vi "Channel Basics Lesson 8.vi"() -> ()   [LabVIEW 2019]
doc: "This VI demonstrates that channels can create cycles among nodes, unlike regular dataflow wires."
uses:
  <extravilib>/ChannelInstances/One Element Stream-i32/Read With Abort.vi
  <extravilib>/ChannelInstances/One Element Stream-i32/Write With Abort.vi
  <extravilib>/ChannelInstances/One Element Stream-i32/Instantiate.vi
  <extravilib>/ChannelInstances/One Element Stream-i32/EndpointRead.vi
  <extravilib>/ChannelInstances/One Element Stream-i32/Endpoint.vi
  <extravilib>/ChannelInstances/One Element Stream-i32.lvlib
panel:
  out "gamma":i32
  out "beta":i32
  out "alpha":i32
  # "Overview: This VI demonstrates that channels can create cycles among nodes, unlike regular dataflow wires.\n\nInstructions:\n1. Open the block diagram. Review the lessons presented there.\n2. Run the VI and observe the values of alpha, beta, and gamma show the results of the integer being passed from loop to loop."
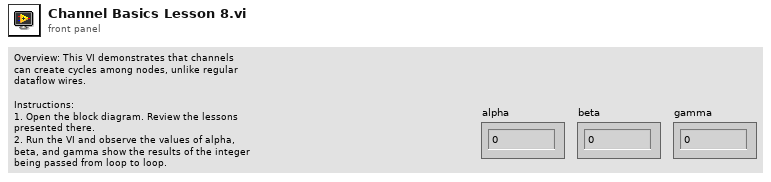
[diagram p1: front panel]
types:
  T1 = typedef "One Element Stream-i32.lvlib/)Channel.ctl" = refnum<queue>
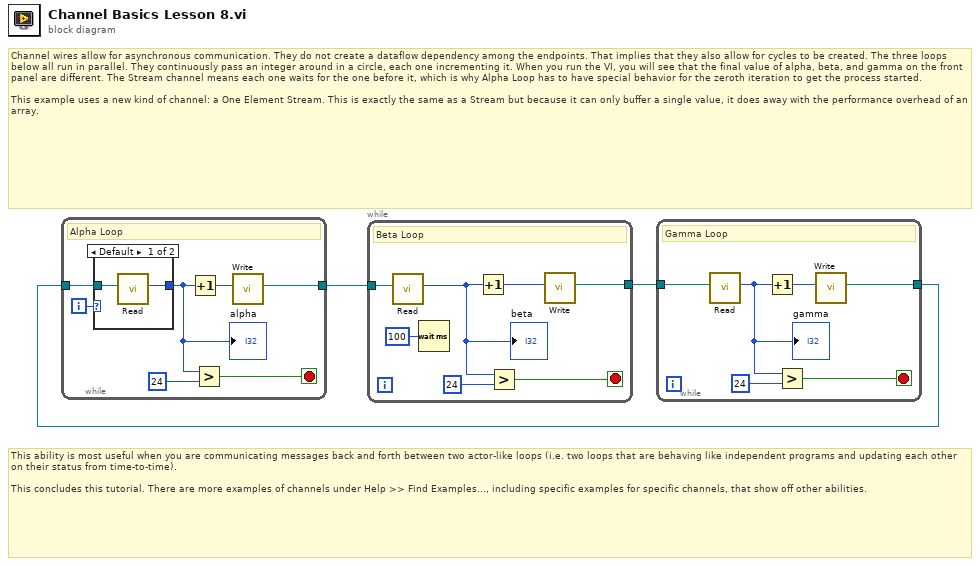
[diagram p0: block diagram]
diagram:
  # "This ability is most useful when you are communicating messages back and forth between two actor-like loops (i.e. two loops that are behaving like independent programs and updating each other on their status from time-to-time).\n\nThis concludes this tutorial. There are more examples of channels under Help >> Find Examples..., including specific examples for specific channels, that show off other abilities."
  # "Channel wires allow for asynchronous communication. They do not create a dataflow dependency among the endpoints. That implies that they also allow for cycles to be created. The three loops below all run in parallel. They continuously pass an integer around in a circle, each one incrementing it. When you run the VI, you will see that the final value of alpha, beta, and gamma on the front panel are different. The Stream channel means each one waits for the one before it, which is why Alpha Loop has to have special behavior for the zeroth iteration to get the process started.\n\nThis example uses a new kind of channel: a One Element Stream. This is exactly the same as a Stream but because it can only buffer a single value, it does away with the performance overhead of an array."
  n1 = while {
    tunnel: [w4] -> w1
    tunnel: w2 -> [w10]
    i -> [w6]
    stop <- w7 stop-if-true
    # "Alpha Loop"
    n2 = case shown="Default" w6 {
      tunnel: w10 -> [w12 _]
      tunnel: [w11 _] -> w9
      frame Default {
        n3 = call <extravilib>:"Read.vi"("channel"=w12) -> ("element"=w11:i32)  [unwired: 7 in, 3 out]
      }
      frame 0 {
      }
    }
    "alpha" <- w9
    n4 = Increment(x=w9) -> (x+1=w5:i32)
    n5 = Greater?(x=w9, y=24) -> (0:w7:bool)
    n6 = call <extravilib>:"Write.vi"("element"=w5) -> ("channel"=w4:T1)  [unwired: 9 in, 1 out]
  }
  n7 = while {
    tunnel: w1 -> [w14]
    tunnel: [w15] -> w3
    stop <- w18 stop-if-true
    # "Beta Loop"
    n8 = call <extravilib>:"Read.vi"("channel"=w14) -> ("element"=w13:i32)  [unwired: 7 in, 3 out]
    "beta" <- w13
    n9 = Wait (ms)(milliseconds to wait=u32 100) -> ()  [unwired: 1 out]
    n10 = Increment(x=w13) -> (x+1=w16:i32)
    n11 = Greater?(x=w13, y=24) -> (0:w18:bool)
    n12 = call <extravilib>:"Write.vi"("element"=w16) -> ("channel"=w15:T1)  [unwired: 9 in, 1 out]
  }
  n13 = while {
    tunnel: w3 -> [w23]
    tunnel: [w20] -> w2
    stop <- w24 stop-if-true
    # "Gamma Loop"
    n14 = call <extravilib>:"Read.vi"("channel"=w23) -> ("element"=w22:i32)  [unwired: 7 in, 3 out]
    "gamma" <- w22
    n15 = Increment(x=w22) -> (x+1=w21:i32)
    n16 = Greater?(x=w22, y=24) -> (0:w24:bool)
    n17 = call <extravilib>:"Write.vi"("element"=w21) -> ("channel"=w20:T1)  [unwired: 9 in, 1 out]
  }
